vi "green puzzle.vi"(10 "Puzzle Color 4":string(xcontrol), 11 "Puzzle Color 5":string(xcontrol)) -> ()   [LabVIEW 2019]
uses:
  Program Files (x86)/National Instruments/LabVIEW 2019/project/EN1Course-master (12)/EN1Course-master/_Subs/ThingWorx/_TW_Subs/TW_XControl.xctl
  Program Files (x86)/National Instruments/LabVIEW 2019/project/EN1Course-master (12)/EN1Course-master/_Subs/ThingWorx/_TW_Subs/Thingworx_Write_string.vi
  <vilib>/httpClient/LabVIEWHTTPClient.lvlib
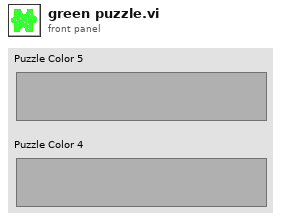
[diagram p1: front panel]
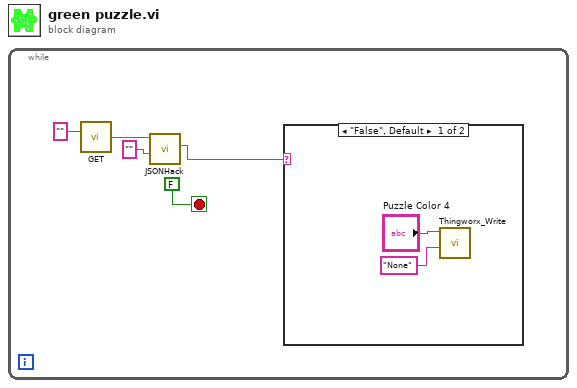
[diagram p0: block diagram]
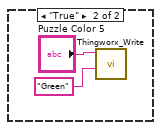
[diagram p2: hidden frame]
diagram:
  n1 = while {
    stop <- FALSE stop-if-true
    n2 = call <vilib>:"GET.vi"("url"="") -> ("body"=w3:string)  [unwired: 11 in, 3 out]
    n3 = call "JSONHack.vi"("search name"="", "JSON in"=w3) -> ("Property (str)"=w1:string)  [unwired: 6 in, 3 out]
    n4 = case shown="\"False\", Default" w1 {
      frame "False", Default {
        n5 = call-poly "Thingworx_Write.vi"("String"="None", "Thingworx"="Puzzle Color 4") -> ()  [unwired: 10 in]
      }
      frame "True" {
        n6 = call-poly "Thingworx_Write.vi"("String"="Green", "Thingworx"="Puzzle Color 5") -> ()  [unwired: 10 in]
      }
    }
  }
